vi "Strafe_Correction.vi"(8 "error in":errorcluster) -> ()   [LabVIEW 2018]
uses:
  <vilib>/Rock Robotics/Network Tables/NT Write Number.vi
panel:
  # ".035"
  # "0"
  # ".002"
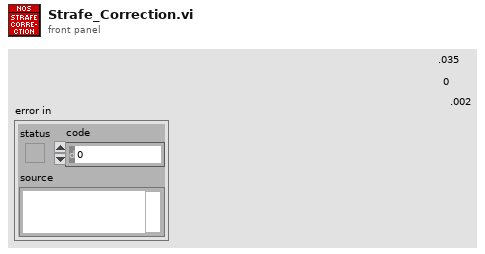
[diagram p1: front panel]
types:
  T1 = cluster{"proportional gain (Kc)":dbl, "integral time (Ti, min)":dbl, "derivative time (Td, min)":dbl}
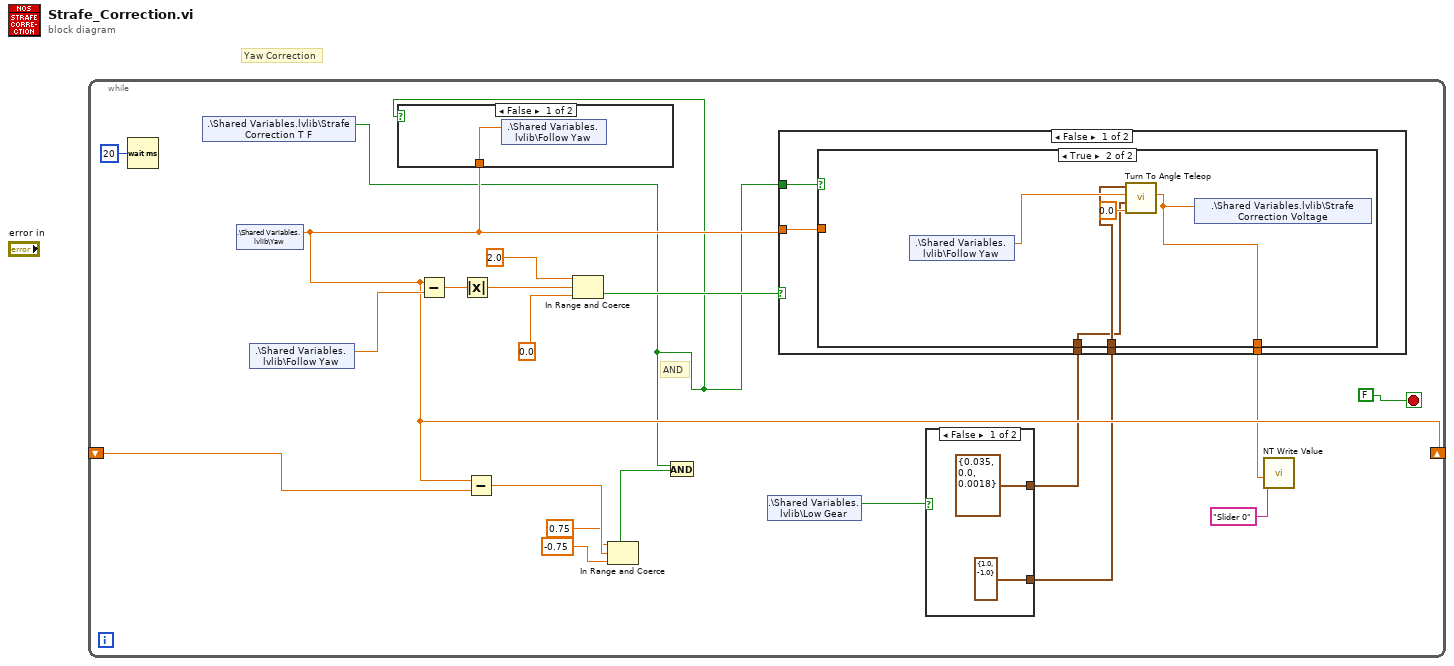
[diagram p0: block diagram]
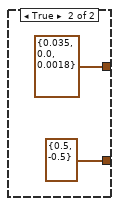
[diagram p2: hidden frame]
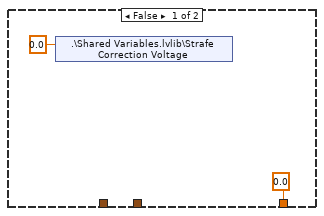
[diagram p4: hidden frame]
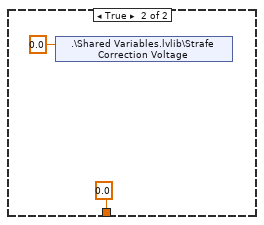
[diagram p5: hidden frame]
diagram:
  # "Yaw Correction"
  n1 = while {
    shift-right: [w12] -> _
    shift-left: _ -> [w11]
    stop <- FALSE stop-if-true
    # "AND"
    n2 = Wait (ms)(milliseconds to wait=u32 20) -> ()  [unwired: 1 out]
    n3 = shared-variable ".\\Shared Variables.lvlib\\Strafe Correction T F"() -> (w2:bool)  [unwired: 1 in, 1 out]
    n4 = shared-variable ".\\Shared Variables.lvlib\\Yaw"() -> (w12:dbl)  [unwired: 1 in, 1 out]
    n5 = shared-variable ".\\Shared Variables.lvlib\\Follow Yaw"() -> (w18:dbl)  [unwired: 1 in, 1 out]
    n6 = case shown="False" w2 {
      tunnel: w12 -> [w25 _]
      frame False {
        n7 = shared-variable ".\\Shared Variables.lvlib\\Follow Yaw"(w25) -> ()  [unwired: 1 in, 1 out]
      }
      frame True {
      }
    }
    n8 = Subtract(x=w12, y=w18) -> (x-y=w15:dbl)
    n9 = Absolute Value(x=w15) -> (abs(x)=w14:dbl)
    n10 = Subtract(x=w12, y=w11) -> (x-y=w10:dbl)
    n11 = In Range and Coerce(upper limit=2.0, x=w14, lower limit=0.0) -> (In Range?=w16:bool)  [unwired: 1 out]
    n12 = In Range and Coerce(upper limit=0.75, x=w10, lower limit=-0.75) -> (In Range?=w1:bool)  [unwired: 1 out]
    n13 = And(x=w2, y=w1) -> ()  [unwired: 1 out]
    n14 = shared-variable ".\\Shared Variables.lvlib\\Low Gear"() -> (w7:bool)  [unwired: 1 in, 1 out]
    n15 = case shown="False" w7 {
      tunnel: [cluster{"output high":dbl, "output low":dbl} {"output high"=1.0, "output low"=-1.0} ("output range") cluster{"output high":dbl, "output low":dbl} {"output high"=0.5, "output low"=-0.5} ("output range")] -> w6
      tunnel: [T1 {"proportional gain (Kc)"=0.035, "integral time (Ti, min)"=0.0, "derivative time (Td, min)"=0.0018} ("PID gains") T1 {"proportional gain (Kc)"=0.035, "integral time (Ti, min)"=0.0, "derivative time (Td, min)"=0.0018} ("PID gains")] -> w5
      frame False {
      }
      frame True {
      }
    }
    n16 = case shown="False" w16 {
      tunnel: w12 -> [w30 _]
      tunnel: w2 -> [w29 _]
      tunnel: w6 -> [w28 _]
      tunnel: w5 -> [w27 _]
      tunnel: [w26 0.0] -> w4
      frame False {
        n17 = case shown="True" w29 {
          tunnel: w30 -> [_ _]
          tunnel: w28 -> [_ w34]
          tunnel: w27 -> [_ w33]
          tunnel: [0.0 w37] -> w26
          frame False {
            n18 = shared-variable ".\\Shared Variables.lvlib\\Strafe Correction Voltage"(0.0 ("Strafe Correction Voltage")) -> ()  [unwired: 1 in, 1 out]
          }
          frame True {
            n19 = shared-variable ".\\Shared Variables.lvlib\\Follow Yaw"() -> (w35:dbl)  [unwired: 1 in, 1 out]
            n20 = call "Turn To Angle Teleop.vi"("Z Axis"=0.0, "PID gains"=w33, "POV"=w35, "output range"=w34) -> ("Adjustment Voltage"=w37:dbl)  [unwired: 7 in]
            n21 = shared-variable ".\\Shared Variables.lvlib\\Strafe Correction Voltage"(w37) -> ()  [unwired: 1 in, 1 out]
          }
        }
      }
      frame True {
        n22 = shared-variable ".\\Shared Variables.lvlib\\Strafe Correction Voltage"(0.0 ("Strafe Correction Voltage")) -> ()  [unwired: 1 in, 1 out]
      }
    }
    n23 = call-poly <vilib>:"NT Write Value.vi"("Numeric"=w4, "Name"="Slider 0") -> ()  [unwired: 9 in, 1 out]
  }
